vi "_CSMQFGV.vi"(6 "Operation":T3, 8 "Error in":errorcluster caption="Error in (no error)", 9 "create if not found? (T)":bool=TRUE, 11 "Name(\"\" to use uuid) in":string) -> (0 "Error out":errorcluster, 1 "Boolean":bool, 2 "Name":string[](array[string]), 3 "Array":T1[](array[typedef]))   [LabVIEW 2014, in "Communicable State Machine.lvlib"]
uses:
  Communicable State Machine.lvlib
  _CSMQFGVOPER.ctl
  _CSMQ.ctl
  Typedef/_Cross JKISM State Data.ctl
  Typedef/_CSM_MSG_TYPE.ctl
  Typedef/_Cross JKISM State Response.ctl
  Typedef/_CSM_MODE.ctl
  Typedef/_CSM Status Change Event Data.ctl
  FGV-BroadcastRegistry/Operation-BroadcastRegistry.ctl
  FGV-BroadcastRegistry/global-CSMQ FGV Change Flag.vi
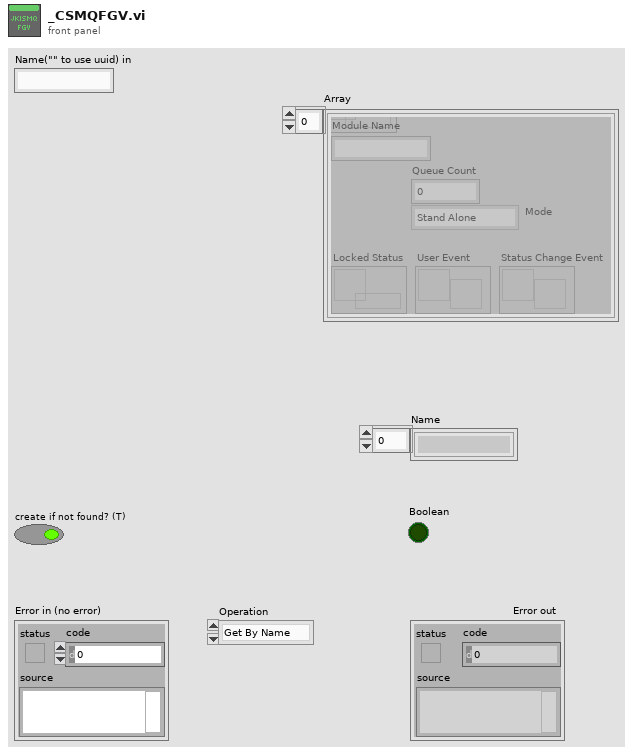
[diagram p1: front panel]
types:
  T1 = typedef "Communicable State Machine.lvlib/_CSMQ.ctl" = cluster{"Module Name":string, "Queue":refnum<queue>, "Locked Status":refnum<data-value>, "Mode":T2, "User Event":refnum<user-event>, "Queue Count":i32, "Status Change Event":refnum<user-event>}
  T2 = typedef "Communicable State Machine.lvlib/_CSM_MODE.ctl" = enum16{"Stand Alone", "CSM", "Action Worker"}
  T3 = typedef "Communicable State Machine.lvlib/_CSMQFGVOPER.ctl" = enum16{"Get By Name", "List", "Check If Name Exists", "Release", "Module Status", "Create Status Event Handler", "Destroy Status Event Handler"}
  T4 = typedef "Communicable State Machine.lvlib/Operation-BroadcastRegistry.ctl" = enum16{"Delete Source Module", "Delete Target Module", "Remove Module", "Register", "Unregister", "Check"}
  T5 = typedef "Communicable State Machine.lvlib/_CSM Status Change Event Data.ctl" = cluster{"ModuleName":string, "Status":string, "Arguments":string}
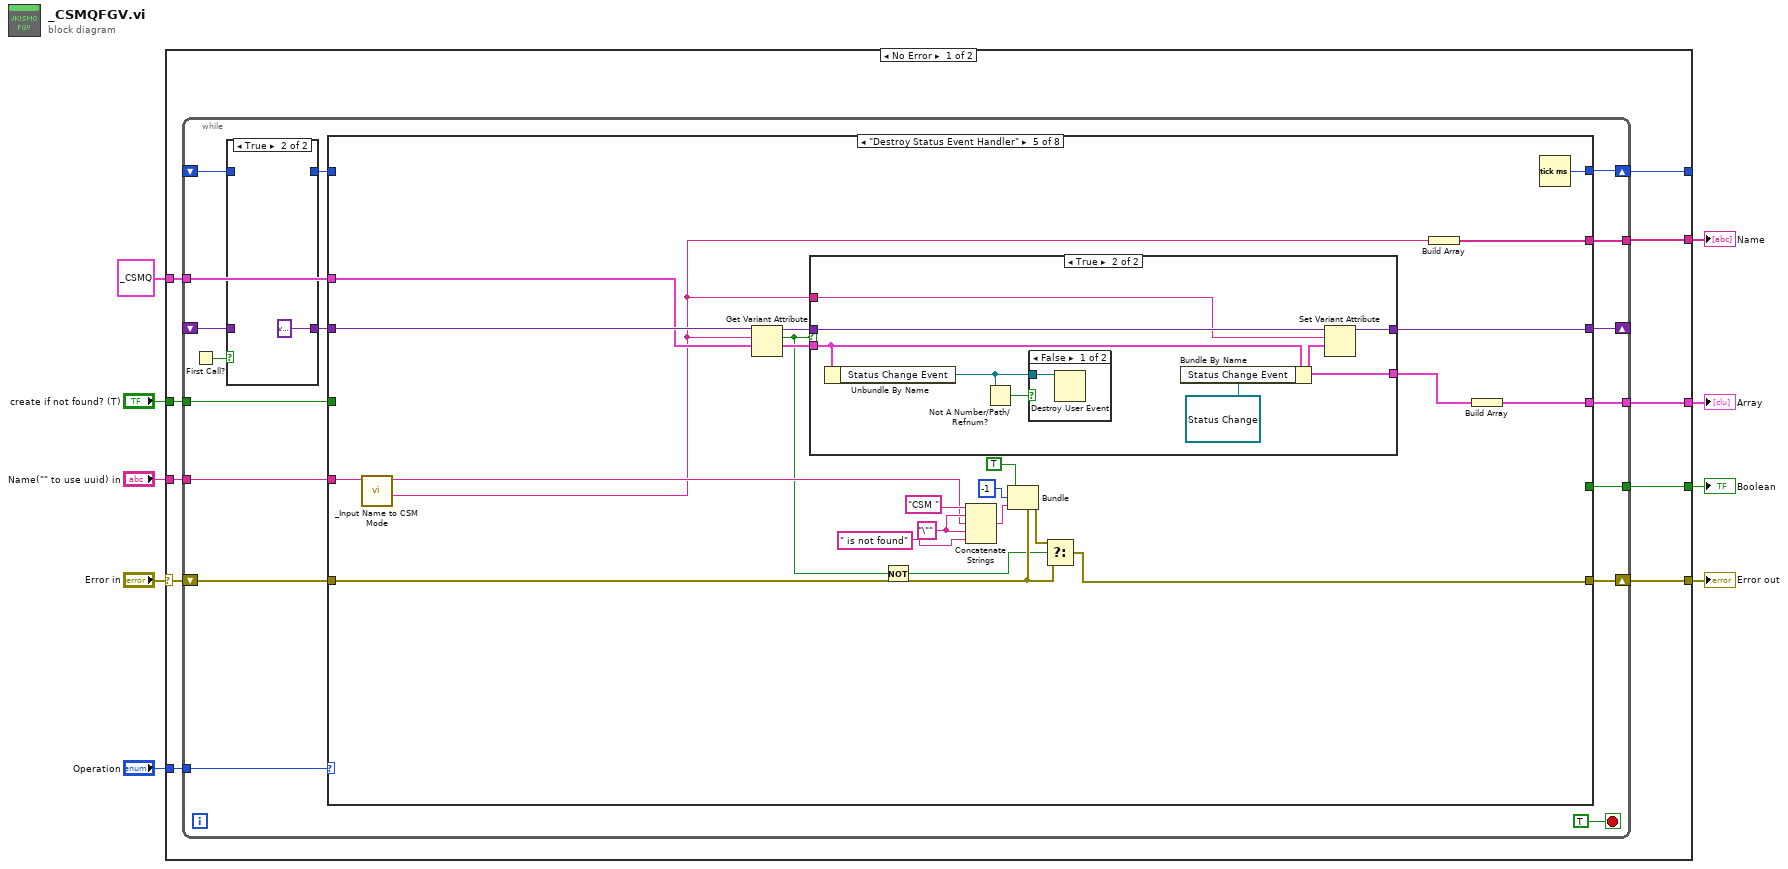
[diagram p0: block diagram]
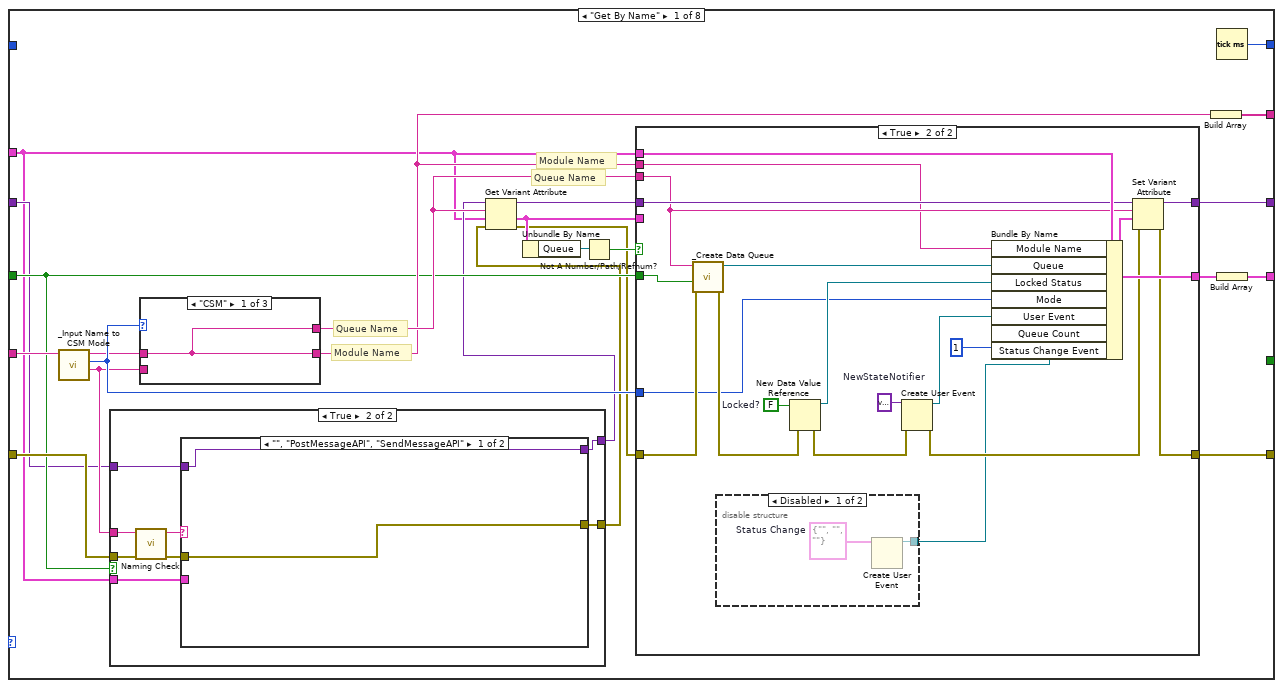
[diagram p3: hidden frame]
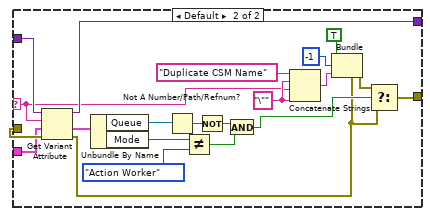
[diagram p5: hidden frame]
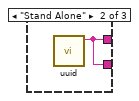
[diagram p6: hidden frame]
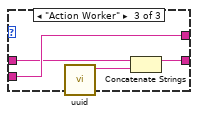
[diagram p7: hidden frame]
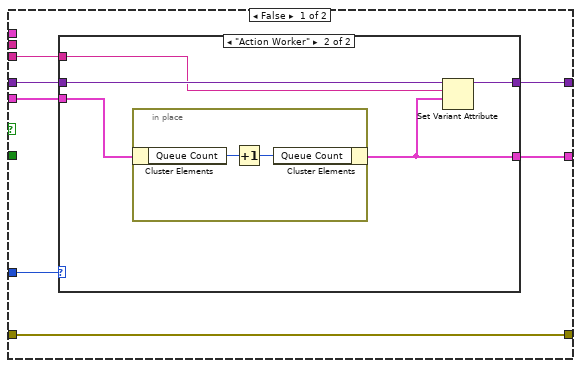
[diagram p8: hidden frame]
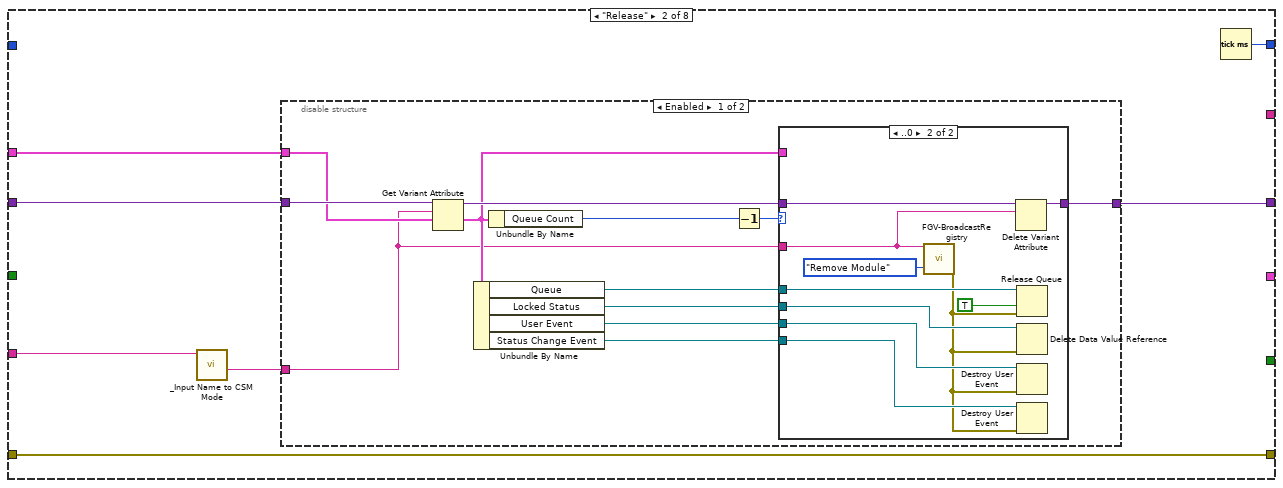
[diagram p11: hidden frame]
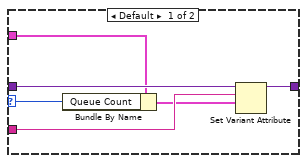
[diagram p12: hidden frame]
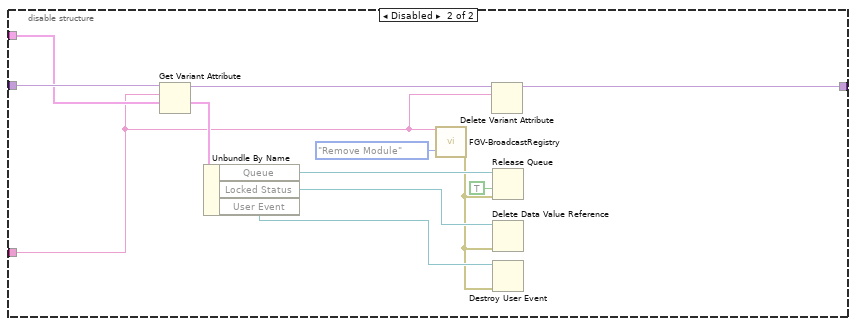
[diagram p13: hidden frame]
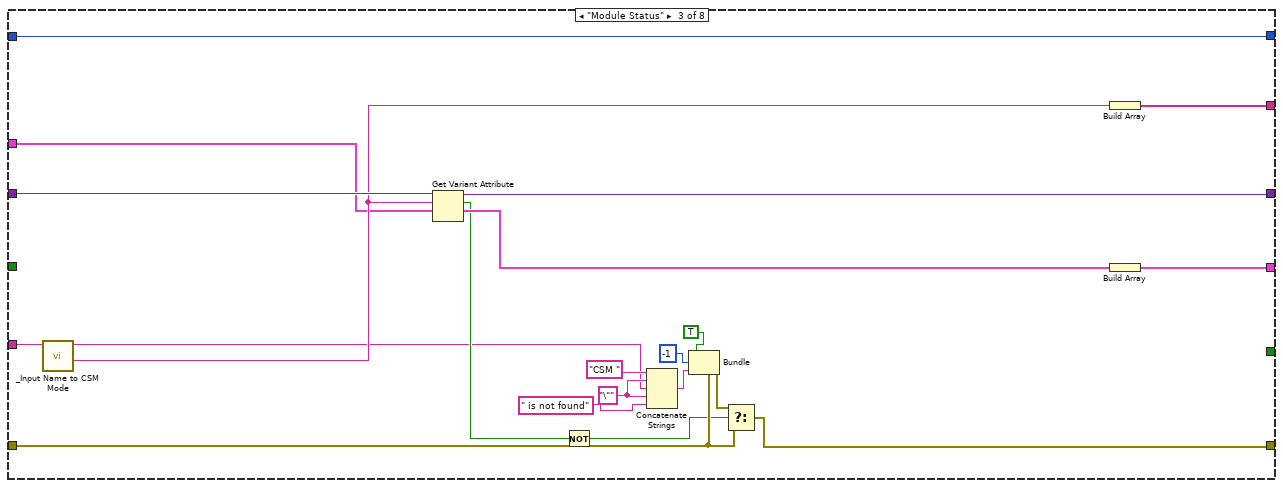
[diagram p14: hidden frame]
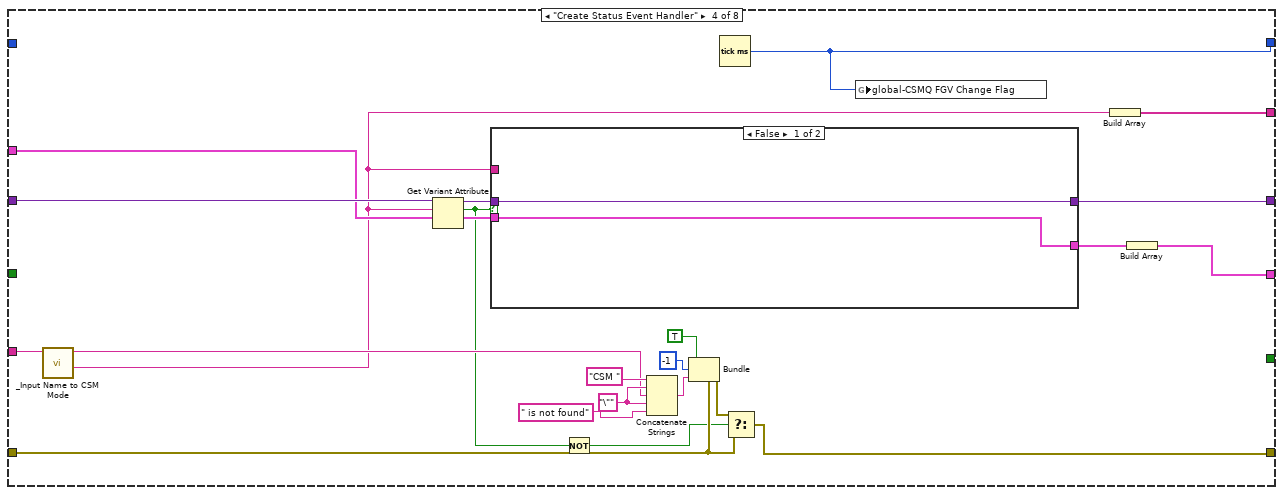
[diagram p15: hidden frame]
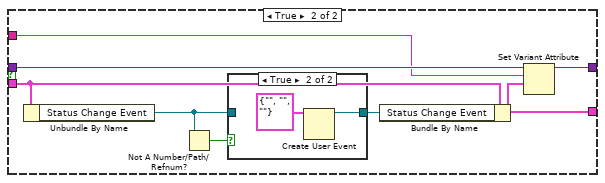
[diagram p16: hidden frame]
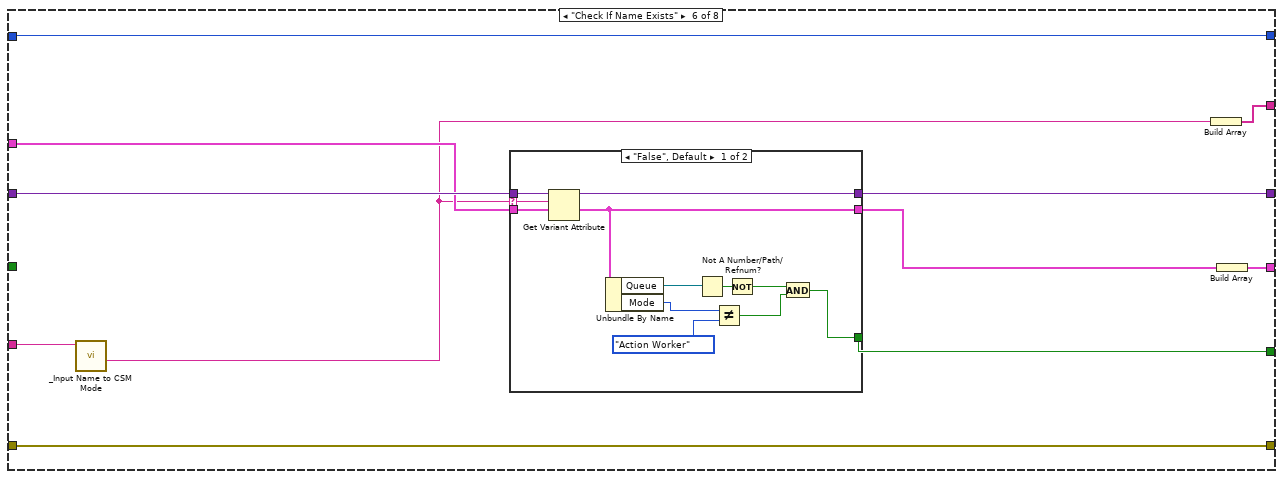
[diagram p20: hidden frame]
diagram:
  n1 = case shown="No Error" "Error in" {
    selector: "Error in" -> [w16 w358]
    tunnel: "Operation" -> [w19 _]
    tunnel: "Name(\"\" to use uuid) in" -> [w18 _]
    tunnel: "create if not found? (T)" -> [w17 _]
    tunnel: [w15 w358] -> w5
    tunnel: [w14 _] -> w4
    tunnel: T1 {"Module Name"="", "Queue"=refnum, "Locked Status"=refnum, "Mode"=enum."Stand Alone", "User Event"=refnum, "Queue Count"=0, "Status Change Event"=refnum} ("CSMQ") -> [w13 _]
    tunnel: [w12 _] -> w2
    tunnel: [w11 _] -> w1
    tunnel: [w10 _] -> _
    frame No Error {
      n2 = while {
        tunnel: w19 -> [w35]
        tunnel: w18 -> [w34]
        tunnel: w17 -> [w33]
        tunnel: [w32] -> w12
        shift-right: [w28] -> _
        shift-left: _ -> [w30]
        shift-right: [w26] -> w15
        shift-left: w16 -> [w27]
        tunnel: [w25] -> w14
        tunnel: w13 -> [w24]
        tunnel: [w23] -> w11
        shift-right: [w22] -> w10
        shift-left: _ -> [w20]
        stop <- TRUE stop-if-true
        n3 = First Call?() -> (First Call?: T/F=w31:bool)
        n4 = case shown="True" w31 {
          tunnel: [w38 variant] -> w29
          tunnel: w30 -> [w38 _]
          tunnel: [w37 _] -> w21
          tunnel: w20 -> [w37 _]
          frame False {
          }
          frame True {
          }
        }
        n5 = case shown="\"Destroy Status Event Handler\"" w35 {
          tunnel: w34 -> [w53 w142 w206 w229 w265 w280 _ _]
          tunnel: w33 -> [w45 _ _ _ _ _ w311 _]
          tunnel: [w55 _ w203 w209 w245 w283 w306 _] -> w32
          tunnel: w29 -> [w44 w145 w207 w230 w266 w288 w319 w357]
          tunnel: [w60 w144 w205 w212 w248 w287 w318 w357] -> w28
          tunnel: w27 -> [w47 w146 w194 w221 w257 w285 w316 w356]
          tunnel: [w56 w146 w191 w219 w255 w285 w315 w356] -> w26
          tunnel: [w54 _ w201 w227 w263 w282 w307 _] -> w25
          tunnel: w24 -> [w42 w143 w199 w226 w262 w284 w317 _]
          tunnel: [_ _ _ _ _ w281 _ _] -> w23
          tunnel: w21 -> [_ _ w200 _ _ w278 w313 w355]
          tunnel: [w48 w140 w200 w208 w244 w278 w313 w355] -> w22
          frame "Get By Name" {
            # "Module Name"
            # "Queue Name"
            # "Module Name"
            # "Queue Name"
            n6 = call "_Input Name to CSM Mode.vi"("String"=w53) -> ("Queue Name"=w46:string, "JKISM Mode"=w52:T2, "String(dup)"=w51:string)  [unwired: 8 in]
            n7 = case shown="True" w45 {
              tunnel: w46 -> [_ w66]
              tunnel: [w64 w72] -> w41
              tunnel: w47 -> [w64 w68]
              tunnel: w44 -> [w63 w71]
              tunnel: [w63 w70] -> w43
              tunnel: w42 -> [_ w69]
              frame False {
              }
              frame True {
                n8 = call "Naming Check.vi"("error in (no error)"=w68, "Name(\"\" to use uuid)"=w66) -> ("error out"=w67:errorcluster, "Name(dup)"=w65:string)  [unwired: 8 in]
                n9 = case shown="\"\", \"PostMessageAPI\", \"SendMessageAPI\"" w65 {
                  selector: w65 -> [_ w75]
                  tunnel: [w73 w95] -> w72
                  tunnel: w67 -> [w73 w78]
                  tunnel: w71 -> [w74 w80]
                  tunnel: [w74 w79] -> w70
                  tunnel: w69 -> [_ w76]
                  frame "", "PostMessageAPI", "SendMessageAPI" {
                  }
                  frame Default {
                    w89 = "\"" ("string")
                    n10 = Get Variant Attribute(Variant=w80, name=w75, default value (empty Variant)=w76, error in=w78) -> (duplicate Variant=w79:variant, value=w82:T1, error out=w77:errorcluster)  [unwired: 1 out]
                    n11 = Unbundle By Name(w82) -> ("Queue"=w83:refnum<queue>, "Mode"=w86:T2)
                    n12 = Not A Number/Path/Refnum?(number/path/refnum=w83) -> (NaN/Path/Refnum?=w84:bool)
                    n13 = Not Equal?(x=w86, y=_CSM_MODE."Action Worker") -> (x != y?=w88:bool)
                    n14 = Not(x=w84) -> (.not. x?=w85:bool)
                    n15 = And(x=w85, y=w88) -> (x .and. y?=w81:bool)
                    n16 = Concatenate Strings("Duplicate CSM Name" ("String to Prepend to source (\"\")"), w89, w75, w89) -> (w90:string)
                    n17 = Bundle(cluster=w77, "status"=TRUE, "code"=-1, "source"=w90) -> (w94:errorcluster)
                    n18 = Select(t=w94, s=w81, f=w77) -> (s? t:f=w95:errorcluster)
                  }
                }
              }
            }
            n19 = case shown="\"CSM\"" w52 {
              tunnel: [w96 w97 w101] -> w50
              tunnel: [w96 w97 w98] -> w49
              tunnel: w51 -> [w96 _ w100]
              tunnel: w46 -> [_ _ w101]
              frame "CSM" {
              }
              frame "Stand Alone" {
                n20 = call "uuid.vi"() -> ("UUID"=w97:string)  [unwired: 11 in]
              }
              frame "Action Worker" {
                n21 = call "uuid.vi"() -> ("UUID"=w99:string)  [unwired: 11 in]
                n22 = Concatenate Strings(w100, w99) -> (w98:string)
              }
            }
            n23 = Get Variant Attribute(Variant=w43, name=w50, default value (empty Variant)=w42, error in=w41) -> (duplicate Variant=w61:variant, value=w59:T1, error out=w40:errorcluster)  [unwired: 1 out]
            n24 = Unbundle By Name(w59) -> ("Queue"=w58:refnum<queue>)
            n25 = Not A Number/Path/Refnum?(number/path/refnum=w58) -> (NaN/Path/Refnum?=w57:bool)
            n26 = case shown="True" w57 {
              tunnel: w45 -> [_ w136]
              tunnel: [w104 w130] -> w62
              tunnel: w50 -> [w102 w120]
              tunnel: w42 -> [_ w133]
              tunnel: w61 -> [w105 w132]
              tunnel: [w106 w131] -> w60
              tunnel: w59 -> [w103 _]
              tunnel: w40 -> [w108 w129]
              tunnel: [w108 w127] -> w56
              tunnel: w52 -> [w107 w122]
              tunnel: w49 -> [_ w119]
              frame False {
                n27 = case shown="\"Action Worker\"" w107 {
                  tunnel: [w110 w114] -> w106
                  tunnel: w105 -> [w110 w115]
                  tunnel: [w109 w111] -> w104
                  tunnel: w103 -> [w109 w112]
                  tunnel: w102 -> [_ w113]
                  frame Default {
                  }
                  frame "Action Worker" {
                    n28 = in-place {
                      n29 = in-place-cluster #1(w112) -> ("Queue Count"=w117:i32)
                      n30 = Increment(x=w117) -> (x+1=w116:i32)
                      n31 = in-place-cluster #1("Queue Count"=w116) -> (w111:T1)
                    }
                    n32 = Set Variant Attribute(Variant=w115, name=w113, value=w111) -> (Variant out=w114:variant)  [unwired: 1 in, 2 out]
                  }
                }
              }
              frame True {
                w126 = variant  # NewStateNotifier
                w137 = FALSE  # Locked?
                n33 = call "_Create Data Queue.vi"("error in (no error)"=w129, "create if not found? (T)"=w136, "Name"=w120) -> ("error out"=w128:errorcluster, "Queue out"=w135:refnum<queue>)  [unwired: 6 in, 1 out]
                n34 = disable-structure shown="Disabled" {
                  disable-tunnel: [w138 _] -> w118
                  frame Disabled {
                    w139 = T5 {"ModuleName"="", "Status"="", "Arguments"=""}  # Status Change
                    n35 = Create User Event(user event datatype=w139) -> (user event=w138:refnum<user-event>)  [unwired: 1 in, 1 out]
                  }
                  frame Enabled {
                  }
                }
                n36 = New Data Value Reference(data value=w137, error in=w128) -> (data value reference=w134:refnum<data-value>, error out=w125:errorcluster)
                n37 = Create User Event(user event datatype=w126, error in=w125) -> (user event=w124:refnum<user-event>, error out=w123:errorcluster)
                n38 = Bundle By Name(cluster=w133, "Module Name"=w119, "Queue"=w135, "Locked Status"=w134, "Mode"=w122, "User Event"=w124, "Queue Count"=1, "Status Change Event"=w118) -> (w130:T1)
                n39 = Set Variant Attribute(Variant=w132, name=w120, value=w130, error in=w123) -> (Variant out=w131:variant, error out=w127:errorcluster)  [unwired: 1 out]
              }
            }
            n40 = Build Array(w49) -> (w54:string[])
            n41 = Tick Count (ms)() -> (millisecond timer value=w48:u32)
            n42 = Build Array(w62) -> (w55:T1[])
          }
          frame "Release" {
            n43 = call "_Input Name to CSM Mode.vi"("String"=w142) -> ("Queue Name"=w141:string)  [unwired: 8 in, 2 out]
            n44 = disable-structure shown="Enabled" {
              disable-tunnel: w145 -> [w155 w183]
              disable-tunnel: [w151 w181] -> w144
              disable-tunnel: w143 -> [w150 w180]
              disable-tunnel: w141 -> [w148 w178]
              frame Enabled {
                n45 = Get Variant Attribute(Variant=w155, name=w148, default value (empty Variant)=w150) -> (duplicate Variant=w152:variant, value=w149:T1)  [unwired: 1 in, 2 out]
                n46 = Unbundle By Name(w149) -> ("Queue"=w158:refnum<queue>, "Locked Status"=w157:refnum<data-value>, "User Event"=w156:refnum<user-event>, "Status Change Event"=w147:refnum<user-event>)
                n47 = Unbundle By Name(w149) -> ("Queue Count"=w154:i32)
                n48 = Decrement(x=w154) -> (x-1=w153:i32)
                n49 = case shown="..0" w153 {
                  selector: w153 -> [w159 _]
                  tunnel: w158 -> [_ w174]
                  tunnel: w157 -> [_ w172]
                  tunnel: w156 -> [_ w171]
                  tunnel: w148 -> [w161 w167]
                  tunnel: w152 -> [w164 w169]
                  tunnel: [w163 w168] -> w151
                  tunnel: w149 -> [w162 _]
                  tunnel: w147 -> [_ w166]
                  frame Default {
                    n50 = Bundle By Name(cluster=w162, "Queue Count"=w159) -> (w160:T1)
                    n51 = Set Variant Attribute(Variant=w164, name=w161, value=w160) -> (Variant out=w163:variant)  [unwired: 1 in, 2 out]
                  }
                  frame ..0 {
                    n52 = call "FGV-BroadcastRegistry.vi"("Source"=w167, "Operation"=Operation-BroadcastRegistry."Remove Module") -> ("Error out"=w165:errorcluster)  [unwired: 11 in, 2 out]
                    n53 = Delete Variant Attribute(6:w167, 7:w169) -> (3:w168:variant)  [unwired: 1 in, 2 out]
                    n54 = Release Queue(queue=w174, force destroy? (F)=TRUE, error in (no error)=w165) -> ()  [unwired: 3 out]
                    n55 = Delete Data Value Reference(data value reference=w172, error in=w165) -> ()  [unwired: 2 out]
                    n56 = Destroy User Event(user event=w171, error in=w165) -> ()  [unwired: 1 out]
                    n57 = Destroy User Event(user event=w166, error in=w165) -> ()  [unwired: 1 out]
                  }
                }
              }
              frame Disabled {
                n58 = Get Variant Attribute(Variant=w183, name=w178, default value (empty Variant)=w180) -> (duplicate Variant=w182:variant, value=w179:T1)  [unwired: 1 in, 2 out]
                n59 = Unbundle By Name(w179) -> ("Queue"=w186:refnum<queue>, "Locked Status"=w185:refnum<data-value>, "User Event"=w184:refnum<user-event>)
                n60 = call "FGV-BroadcastRegistry.vi"("Source"=w178, "Operation"=Operation-BroadcastRegistry."Remove Module") -> ("Error out"=w175:errorcluster)  [unwired: 11 in, 2 out]
                n61 = Delete Variant Attribute(6:w178, 7:w182) -> (3:w181:variant)  [unwired: 1 in, 2 out]
                n62 = Release Queue(queue=w186, force destroy? (F)=TRUE, error in (no error)=w175) -> ()  [unwired: 3 out]
                n63 = Delete Data Value Reference(data value reference=w185, error in=w175) -> ()  [unwired: 2 out]
                n64 = Destroy User Event(user event=w184, error in=w175) -> ()  [unwired: 1 out]
              }
            }
            n65 = Tick Count (ms)() -> (millisecond timer value=w140:u32)
          }
          frame "Module Status" {
            w195 = "\"" ("string")
            n66 = call "_Input Name to CSM Mode.vi"("String"=w206) -> ("Queue Name"=w202:string, "String(dup)"=w189:string)  [unwired: 8 in, 1 out]
            n67 = Get Variant Attribute(Variant=w207, name=w202, default value (empty Variant)=w199) -> (duplicate Variant=w205:variant, found=w193:bool, value=w204:T1)  [unwired: 1 in, 1 out]
            n68 = Not(x=w193) -> (.not. x?=w192:bool)
            n69 = Concatenate Strings("CSM " ("String to Prepend to source (\"\")"), w195, w189, w195, " is not found" ("string")) -> (w196:string)
            n70 = Bundle(cluster=w194, "status"=TRUE, "code"=-1, "source"=w196) -> (w198:errorcluster)
            n71 = Select(t=w198, s=w192, f=w194) -> (s? t:f=w191:errorcluster)
            n72 = Build Array(w202) -> (w201:string[])
            n73 = Build Array(w204) -> (w203:T1[])
          }
          frame "Create Status Event Handler" {
            w222 = "\"" ("string")
            n74 = call "_Input Name to CSM Mode.vi"("String"=w229) -> ("Queue Name"=w211:string, "String(dup)"=w217:string)  [unwired: 8 in, 1 out]
            n75 = Get Variant Attribute(Variant=w230, name=w211, default value (empty Variant)=w226) -> (duplicate Variant=w213:variant, found=w214:bool, value=w228:T1)  [unwired: 1 in, 1 out]
            n76 = case shown="False" w214 {
              tunnel: w228 -> [w231 w235]
              tunnel: w213 -> [w232 w240]
              tunnel: [w232 w239] -> w212
              tunnel: w211 -> [_ w238]
              tunnel: [w231 w233] -> w210
              frame False {
              }
              frame True {
                n77 = Unbundle By Name(w235) -> ("Status Change Event"=w236:refnum<user-event>)
                n78 = Not A Number/Path/Refnum?(number/path/refnum=w236) -> (NaN/Path/Refnum?=w237:bool)
                n79 = case shown="True" w237 {
                  tunnel: w236 -> [w241 _]
                  tunnel: [w241 w242] -> w234
                  frame False {
                  }
                  frame True {
                    n80 = Create User Event(user event datatype=T5 {"ModuleName"="", "Status"="", "Arguments"=""} ("Status Message")) -> (user event=w242:refnum<user-event>)  [unwired: 1 in, 1 out]
                  }
                }
                n81 = Bundle By Name(cluster=w235, "Status Change Event"=w234) -> (w233:T1)
                n82 = Set Variant Attribute(Variant=w240, name=w238, value=w233) -> (Variant out=w239:variant)  [unwired: 1 in, 2 out]
              }
            }
            n83 = Not(x=w214) -> (.not. x?=w220:bool)
            n84 = Concatenate Strings("CSM " ("String to Prepend to source (\"\")"), w222, w217, w222, " is not found" ("string")) -> (w223:string)
            n85 = Bundle(cluster=w221, "status"=TRUE, "code"=-1, "source"=w223) -> (w225:errorcluster)
            n86 = Tick Count (ms)() -> (millisecond timer value=w208:u32)
            n87 = Select(t=w225, s=w220, f=w221) -> (s? t:f=w219:errorcluster)
            n88 = global write "global-CSMQ FGV Change Flag.vi" "global-CSMQ FGV Change Flag"(w208) -> ()
            n89 = Build Array(w211) -> (w227:string[])
            n90 = Build Array(w210) -> (w209:T1[])
          }
          frame "Destroy Status Event Handler" {
            w258 = "\"" ("string")
            n91 = call "_Input Name to CSM Mode.vi"("String"=w265) -> ("Queue Name"=w247:string, "String(dup)"=w253:string)  [unwired: 8 in, 1 out]
            n92 = Get Variant Attribute(Variant=w266, name=w247, default value (empty Variant)=w262) -> (duplicate Variant=w249:variant, found=w250:bool, value=w264:T1)  [unwired: 1 in, 1 out]
            n93 = case shown="True" w250 {
              tunnel: w264 -> [w267 w271]
              tunnel: w249 -> [w268 w276]
              tunnel: [w268 w275] -> w248
              tunnel: w247 -> [_ w274]
              tunnel: [w267 w270] -> w246
              frame False {
              }
              frame True {
                n94 = Unbundle By Name(w271) -> ("Status Change Event"=w272:refnum<user-event>)
                n95 = Not A Number/Path/Refnum?(number/path/refnum=w272) -> (NaN/Path/Refnum?=w273:bool)
                n96 = case shown="False" w273 {
                  tunnel: w272 -> [w277 _]
                  frame False {
                    n97 = Destroy User Event(user event=w277) -> ()  [unwired: 1 in, 1 out]
                  }
                  frame True {
                  }
                }
                n98 = Bundle By Name(cluster=w271, "Status Change Event"=refnum<user-event> refnum) -> (w270:T1)
                n99 = Set Variant Attribute(Variant=w276, name=w274, value=w270) -> (Variant out=w275:variant)  [unwired: 1 in, 2 out]
              }
            }
            n100 = Not(x=w250) -> (.not. x?=w256:bool)
            n101 = Concatenate Strings("CSM " ("String to Prepend to source (\"\")"), w258, w253, w258, " is not found" ("string")) -> (w259:string)
            n102 = Bundle(cluster=w257, "status"=TRUE, "code"=-1, "source"=w259) -> (w261:errorcluster)
            n103 = Select(t=w261, s=w256, f=w257) -> (s? t:f=w255:errorcluster)
            n104 = Build Array(w247) -> (w263:string[])
            n105 = Build Array(w246) -> (w245:T1[])
            n106 = Tick Count (ms)() -> (millisecond timer value=w244:u32)
          }
          frame "Check If Name Exists" {
            n107 = call "_Input Name to CSM Mode.vi"("String"=w280) -> ("Queue Name"=w279:string)  [unwired: 8 in, 2 out]
            n108 = case shown="\"False\", Default" w279 {
              selector: w279 -> [w297 _]
              tunnel: w288 -> [w300 w303]
              tunnel: [w299 w303] -> w287
              tunnel: [w296 w301] -> w286
              tunnel: w284 -> [w298 w301]
              tunnel: [w292 TRUE] -> w281
              frame "False", Default {
                n109 = Get Variant Attribute(Variant=w300, name=w297, default value (empty Variant)=w298) -> (duplicate Variant=w299:variant, value=w296:T1)  [unwired: 1 in, 2 out]
                n110 = Unbundle By Name(w296) -> ("Queue"=w295:refnum<queue>, "Mode"=w291:T2)
                n111 = Not A Number/Path/Refnum?(number/path/refnum=w295) -> (NaN/Path/Refnum?=w294:bool)
                n112 = Not Equal?(x=w291, y=_CSM_MODE."Action Worker") -> (x != y?=w289:bool)
                n113 = Not(x=w294) -> (.not. x?=w293:bool)
                n114 = And(x=w293, y=w289) -> (x .and. y?=w292:bool)
              }
              frame "" {
              }
            }
            n115 = Build Array(w279) -> (w282:string[])
            n116 = Build Array(w286) -> (w283:T1[])
          }
          frame "List" {
            n117 = feedback-in #2(w313) -> ()
            n118 = feedback #2() -> (w314:u32)  [unwired: 1 in]
            n119 = feedback #3() -> (w312:bool)  [unwired: 1 in]
            n120 = feedback-in #3(w311) -> ()
            n121 = Not Equal?(x=w313, y=w314) -> (x != y?=w309:bool)
            n122 = Not Equal?(x=w311, y=w312) -> (x != y?=w310:bool)
            n123 = Or(x=w309, y=w310) -> (x .or. y?=w308:bool)
            n124 = feedback #4() -> (w304:string[])  [unwired: 1 in]
            n125 = feedback #5() -> (w305:T1[])  [unwired: 1 in]
            n126 = case shown="True" w308 {
              tunnel: w319 -> [w321 w336]
              tunnel: [w321 w335] -> w318
              tunnel: w317 -> [_ w333]
              tunnel: [w322 w329] -> w307
              tunnel: [w323 w328] -> w306
              tunnel: w316 -> [w320 w326]
              tunnel: [w320 w325] -> w315
              tunnel: w311 -> [_ w324]
              tunnel: w305 -> [w323 _]
              tunnel: w304 -> [w322 _]
              frame False {
              }
              frame True {
                n127 = disable-structure shown="Enabled" {
                  disable-tunnel: w333 -> [w354 _]
                  disable-tunnel: [w353 _] -> w332
                  frame Disabled {
                    n128 = Build Array(w354) -> (w353:T1[])
                  }
                  frame Enabled {
                  }
                }
                n129 = Get Variant Attribute(Variant=w336, error in=w326) -> (duplicate Variant=w335:variant, names=w330:string[], values=w334:variant[], error out=w327:errorcluster)  [unwired: 2 in]
                n130 = Variant To Data(error in=w327, type=w332, Variant=w334) -> (data=w331:T1[], error out=w325:errorcluster)
                n131 = for {
                  tunnel: w331 -> [w349] mode=indexing
                  tunnel: w330 -> [w340] mode=indexing
                  tunnel: [w340] -> w329 mode=indexing if=w341
                  tunnel: [w349] -> w328 mode=indexing if=w341
                  tunnel: w324 -> [w342]
                  n132 = Unbundle By Name(w349) -> ("Queue"=w348:refnum<queue>, "Mode"=w344:T2)
                  n133 = case shown="Default" w344 {
                    tunnel: [w350 TRUE] -> w343
                    tunnel: w342 -> [w351 _]
                    frame "Stand Alone" {
                      n134 = Not(x=w351) -> (.not. x?=w350:bool)
                    }
                    frame Default {
                    }
                  }
                  n135 = Not A Number/Path/Refnum?(number/path/refnum=w348) -> (NaN/Path/Refnum?=w347:bool)
                  n136 = Not(x=w347) -> (.not. x?=w345:bool)
                  n137 = Match Pattern(string=w340, regular expression="^-") -> (offset past match=w338:i32)  [unwired: 1 in, 3 out]
                  n138 = And(x=w345, y=w343) -> (x .and. y?=w346:bool)
                  n139 = Less Than 0?(x=w338) -> (x < 0?=w337:bool)
                  n140 = And(x=w337, y=w346) -> (x .and. y?=w341:bool)
                }
              }
            }
            n141 = feedback-in #4(w307) -> ()
            n142 = feedback-in #5(w306) -> ()
          }
          frame Default {
          }
        }
      }
    }
    frame Error {
    }
  }
  "Error out" <- w5
  "Name" <- w4
  "Array" <- w2
  "Boolean" <- w1
